vi "Target System.vi"(9 "Buttons":T1, 10 "Axes":T2, 11 "Target Info":T3(array[cluster])) -> ()   [LabVIEW 2011]
uses:
  <vilib>/Rock Robotics/WPI/Joystick/WPI_JoystickButtonState.ctl
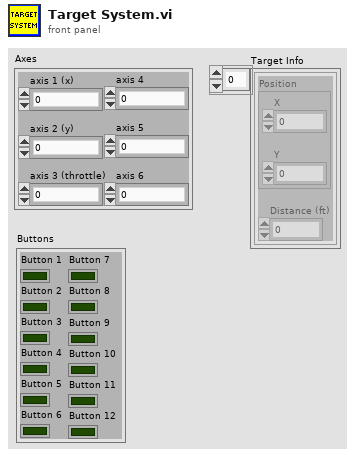
[diagram p1: front panel]
types:
  T1 = typedef "WPI_JoystickButtonState.ctl" = cluster{"Button 1":bool, "Button 2":bool, "Button 3":bool, "Button 4":bool, "Button 5":bool, "Button 6":bool, "Button 7":bool, "Button 8":bool, "Button 9":bool, "Button 10":bool, "Button 11":bool, "Button 12":bool}
  T2 = cluster{"axis 1 (x)":dbl, "axis 2 (y)":dbl, "axis 3 (throttle)":dbl, "axis 4":dbl, "axis 5":dbl, "axis 6":dbl}
  T3 = cluster{"Position":cluster{"X":dbl, "Y":dbl}, "Distance (ft)":dbl}[]
  T4 = typedef "WPI_MotorControlDeviceRef.ctl" = cluster{"DeviceStatus":errorcluster, "Type":enum16{"PWM", "CAN"}, "PWM":cluster{"Digital Module":T5, "PWM Channel":T6, "DeadBand":T7}, "CAN":cluster{"Device Number":u8, "Control Mode":T8, "Semaphore":T9, "Max Vout":dbl}, "Invert":bool, "TransformRef":T10, "InvTransformRef":T10}
  T5 = typedef "FPGA_TypedefDigitalModule.ctl" = enum16{"Digital Module 1", "Digital Module 2"}
  T6 = typedef "FPGA_DIOPWMChannel.ctl" = enum8{"PWM 1", "PWM 2", "PWM 3", "PWM 4", "PWM 5", "PWM 6", "PWM 7", "PWM 8", "PWM 9", "PWM 10", "Invalid"}
  T7 = typedef "WPI_PWMDeadband.ctl" = cluster{"Name":string, "maxPositivePwm":i32, "minPositivePwm":i32, "centerPwm":i32, "maxNegativePwm":i32, "minNegativePwm":i32, "angularRange":u16}
  T8 = typedef "WPI_CANJaguar_ControlMode.ctl" = enum8{"Percent VBus", "Current", "Speed", "Position", "Voltage"}
  T9 = typedef "Semaphore RefNum" = refnum<k1>
  T10 = typedef "WPI_PWMTransform_ConPane.ctl" = refnum<vi>
  T11 = typedef "WPI_ServoDeviceRef.ctl" = cluster{"DeviceStatus":errorcluster, "Digital Module":T5, "PWM Channel":T6, "DeadBand":T7}
  T12 = cluster{"Position":cluster{"X":dbl, "Y":dbl}, "Distance (ft)":dbl}
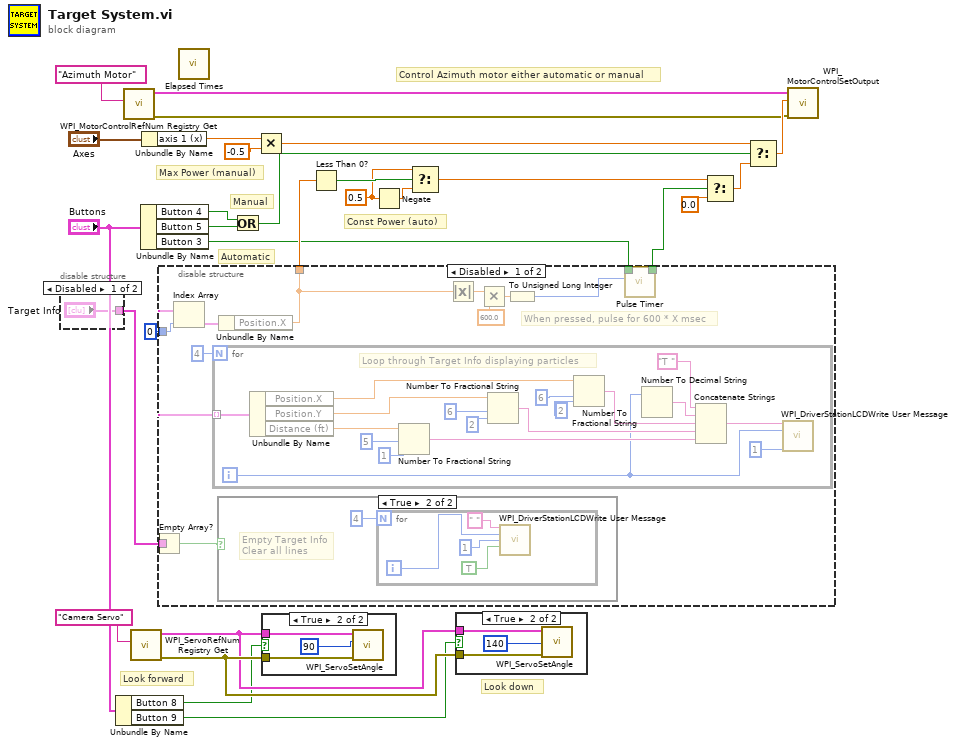
[diagram p0: block diagram]
diagram:
  w11 = 0.5
  # "Look down"
  # "Look forward"
  # "Const Power (auto)"
  # "Max Power (manual)"
  # "Manual"
  # "Automatic"
  # "Control Azimuth motor either automatic or manual"
  n1 = disable-structure shown="Disabled" {
    disable-tunnel: ["Target Info" _] -> w18
    frame Disabled {
    }
    frame Enabled {
    }
  }
  n2 = Unbundle By Name("Buttons") -> ("Button 8"=w1:bool, "Button 9"=w2:bool)
  n3 = call <vilib>:"WPI_MotorControlRefNum Registry Get.vi"("refnum name"="Azimuth Motor") -> ("error out"=w5:errorcluster, "MotorControlDevRef"=w27:T4)  [unwired: 9 in]
  n4 = call <vilib>:"WPI_ServoRefNum Registry Get.vi"("refnum name"="Camera Servo") -> ("error out"=w4:errorcluster, "ServoDeviceRef"=w3:T11)  [unwired: 9 in]
  n5 = Unbundle By Name("Buttons") -> ("Button 4"=w25:bool, "Button 5"=w24:bool, "Button 3"=w9:bool)
  n6 = Unbundle By Name("Axes") -> ("axis 1 (x)"=w21:dbl)
  n7 = disable-structure shown="Disabled" {
    disable-tunnel: w18 -> [w40 _]
    disable-tunnel: 0 ("index") -> [w38 _]
    disable-tunnel: [w35 _] -> w10
    disable-tunnel: w9 -> [w34 _]
    disable-tunnel: [w32 _] -> w8
    frame Disabled {
      # "When pressed, pulse for 600 * X msec"
      n8 = Empty Array?(array=w40) -> (empty?=w30:bool)
      n9 = Index Array(array=w40, index=w38) -> (element=w41:T12)
      n10 = for {
        N: 4 -> [_]
        tunnel: w40 -> [w64] mode=indexing
        i -> [w47]
        # "Loop through Target Info displaying particles"
        n11 = Unbundle By Name(w64) -> ("Position.X"=w53:dbl, "Position.Y"=w52:dbl, "Distance (ft)"=w51:dbl)
        n12 = Number To Fractional String(number=w51, width (-)=i16 5, precision (6)=i16 1) -> (F-format string=w62:string)  [unwired: 1 in]
        n13 = Number To Fractional String(number=w52, width (-)=i16 6, precision (6)=i16 2) -> (F-format string=w61:string)  [unwired: 1 in]
        n14 = Number To Fractional String(number=w53, width (-)=i16 6, precision (6)=i16 2) -> (F-format string=w55:string)  [unwired: 1 in]
        n15 = Number To Decimal String(number=w47) -> (decimal integer string=w48:string)  [unwired: 1 in]
        n16 = Concatenate Strings("T " ("string"), w48, w55, w61, w62) -> (w54:string)
        n17 = call <vilib>:"WPI_DriverStationLCDWrite User Message.vi"("line text"=w54, "line"=w47, "starting column"=i8 1) -> ()  [unwired: 12 in, 1 out]
      }
      n18 = case shown="True" w30 {
        frame False {
        }
        frame True {
          # "Empty Target Info\nClear all lines"
          n19 = for {
            N: 4 -> [_]
            i -> [w44]
            n20 = call <vilib>:"WPI_DriverStationLCDWrite User Message.vi"("line text"=" ", "line"=w44, "starting column"=i8 1, "clear line before write (T)"=TRUE) -> ()  [unwired: 11 in, 1 out]
          }
        }
      }
      n21 = Unbundle By Name(w41) -> ("Position.X"=w35:dbl)
      n22 = Absolute Value(x=w35) -> (abs(x)=w37:dbl)
      n23 = Multiply(x=w37, y=600.0) -> (x*y=w36:dbl)
      n24 = To Unsigned Long Integer(number=w36) -> (unsigned 32bit integer=w33:u32)
      n25 = call "Pulse Timer.vi"("Time"=w33, "Start"=w34) -> ("Timeout"=w32:bool)  [unwired: 8 in, 1 out]
    }
    frame Enabled {
    }
  }
  n26 = call "Elapsed Times.vi"() -> ()  [unwired: 3 in, 1 out]
  n27 = Or(x=w25, y=w24) -> (x .or. y?=w16:bool)
  n28 = Multiply(x=w21, y=-0.5) -> (x*y=w15:dbl)
  n29 = case shown="True" w1 {
    tunnel: w3 -> [_ w67]
    tunnel: w4 -> [_ w66]
    frame False {
    }
    frame True {
      n30 = call <vilib>:"WPI_ServoSetAngle.vi"("error in (no error)"=w66, "Angle"=u16 90 ("t"), "ServoDeviceRef"=w67) -> ()  [unwired: 7 in, 2 out]
    }
  }
  n31 = Less Than 0?(x=w10) -> (x < 0?=w14:bool)
  n32 = Negate(x=w11) -> (-x=w12:dbl)
  n33 = Select(t=w11, s=w14, f=w12) -> (s? t:f=w13:dbl)
  n34 = case shown="True" w2 {
    tunnel: w4 -> [_ w70]
    tunnel: w3 -> [_ w68]
    frame False {
    }
    frame True {
      n35 = call <vilib>:"WPI_ServoSetAngle.vi"("error in (no error)"=w70, "Angle"=u16 140 ("t"), "ServoDeviceRef"=w68) -> ()  [unwired: 7 in, 2 out]
    }
  }
  n36 = Select(t=w13, s=w8, f=0.0) -> (s? t:f=w20:dbl)
  n37 = Select(t=w15, s=w16, f=w20) -> (s? t:f=w19:dbl)
  n38 = call <vilib>:"WPI_MotorControlSetOutput.vi"("error in (no error)"=w5, "Output"=w19, "MotorControlDevRef"=w27) -> ()  [unwired: 7 in, 2 out]
